vi "Introspection Core.vi"(8 "error in (no error)":errorcluster, 11 "CS++Motor in":refnum<class "CS++Motor.lvclass">) -> (0 "error out":errorcluster, 2 "CS++Messages":refnum<class "Message.lvclass">[](array[class]), 3 "CS++Motor out":refnum<class "CS++Motor.lvclass">)   [LabVIEW 2016, in "CS++Motor.lvlib" / "CS++Motor.lvclass"]
doc: "This vi delivers a list with all messages this actor reacts to. \n\nNote that all inherited classes have to overwrite it."
uses:
  CS++Motor.lvclass
  <vilib>/ActorFramework/Message/Message.lvclass
  CS++Motor Messages/Move Msg/Move Msg.lvclass
  C:/Program Files (x86)/National Instruments/LabVIEW 2016/vi.lib/ActorFramework/Message/Message.lvclass
  CS++Motor Messages/ReferenceMove Msg/ReferenceMove Msg.lvclass
  CS++Motor Messages/AbortAllMovements Msg/AbortAllMovements Msg.lvclass
  CS++Motor Messages/Update_Error Msg/Update_Error Msg.lvclass
  CS++Motor Messages/Update_Moving Msg/Update_Moving Msg.lvclass
  CS++Motor Messages/Update_RawActPosition Msg/Update_RawActPosition Msg.lvclass
  CS++Motor Messages/Update_Referenced Msg/Update_Referenced Msg.lvclass
  CS++Motor Messages/StopMovement Msg/StopMovement Msg.lvclass
  CSPP_Core/Actors/CS++DeviceActor/CS++DeviceActor.lvclass
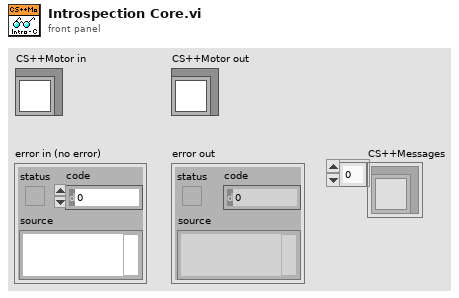
[diagram p1: front panel]
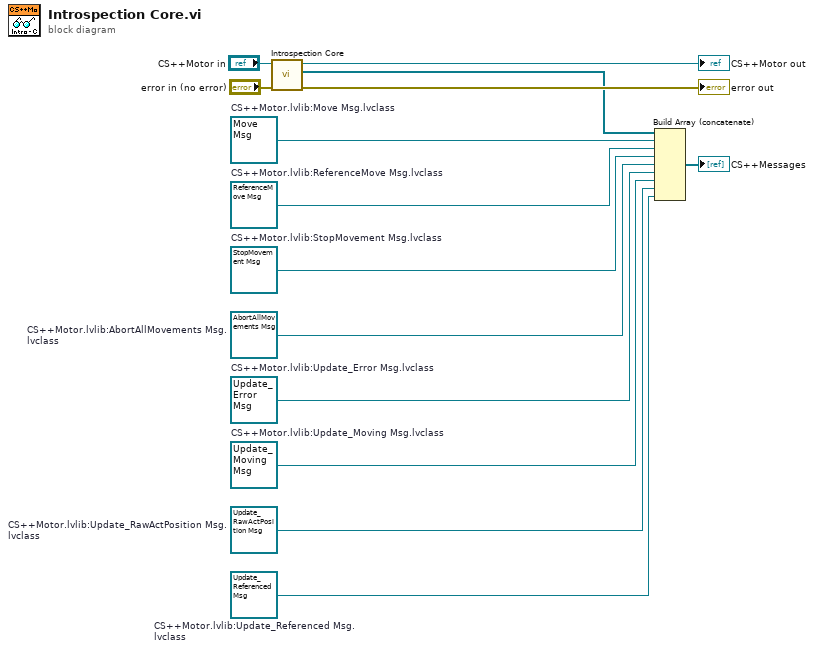
[diagram p0: block diagram]
diagram:
  w1 = refnum<class "StopMovement Msg.lvclass"> refnum  # CS++Motor.lvlib:StopMovement Msg.lvclass
  w3 = refnum<class "Update_Referenced Msg.lvclass"> refnum  # CS++Motor.lvlib:Update_Referenced Msg.lvclass
  w4 = refnum<class "Update_RawActPosition Msg.lvclass"> refnum  # CS++Motor.lvlib:Update_RawActPosition Msg.lvclass
  w5 = refnum<class "Update_Moving Msg.lvclass"> refnum  # CS++Motor.lvlib:Update_Moving Msg.lvclass
  w6 = refnum<class "Update_Error Msg.lvclass"> refnum  # CS++Motor.lvlib:Update_Error Msg.lvclass
  w2 = refnum<class "AbortAllMovements Msg.lvclass"> refnum  # CS++Motor.lvlib:AbortAllMovements Msg.lvclass
  w7 = refnum<class "ReferenceMove Msg.lvclass"> refnum  # CS++Motor.lvlib:ReferenceMove Msg.lvclass
  w8 = refnum<class "Move Msg.lvclass"> refnum  # CS++Motor.lvlib:Move Msg.lvclass
  n1 = call-parent "Introspection Core.vi"("error in (no error)"="error in (no error)", "CS++DeviceActor in"="CS++Motor in") -> ("error out"=→"error out":errorcluster, "CS++Messages"=w10:refnum<class "Message.lvclass">[], "CS++DeviceActor out"=→"CS++Motor out":refnum<class "CS++Motor.lvclass">)  [unwired: 7 in]
  n2 = Build Array (concatenate)(w10, w8, w7, w1, w2, w6, w5, w4, w3) -> (→"CS++Messages":refnum<class "Message.lvclass">[])
